vi "Baseplate Locate.vi"() -> ()   [LabVIEW 2020]
uses:
  Classes/Workspace/Workspace.ctl
  Classes/Workspace/Carrier Tray/Assembly Tray.lvclass
  Classes/Controller/Controller.lvclass
  Classes/Routine/Pick and Place/Pick and Place.lvclass
  Classes/Workspace/Fixture.lvclass
panel:
  out "Workspace":T1
  out "Array":dbl[](array[numeric])
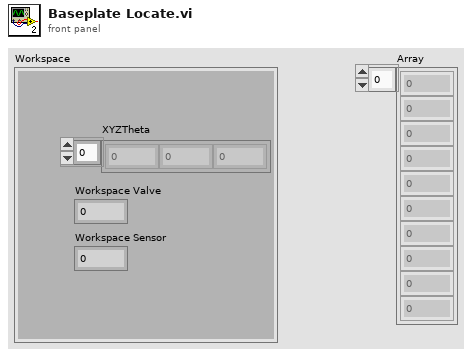
[diagram p1: front panel]
types:
  T1 = typedef "Fixture.lvclass/Workspace.ctl" = cluster{"XYZTheta":dbl[], "Workspace Valve":i32, "Workspace Sensor":i32}
  T2 = typedef "Controller.lvclass/Controllers.ctl" = cluster{"I-O.lvclass":refnum<class "I-O.lvclass">, "Dispenser.lvclass":refnum<class "Dispenser.lvclass">, "Gantry":refnum<k24>}
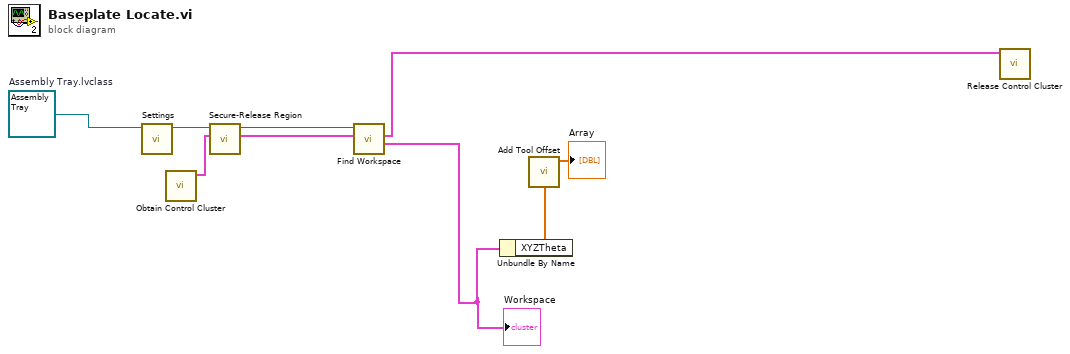
[diagram p0: block diagram]
diagram:
  w9 = refnum<class "Assembly Tray.lvclass"> refnum  # Assembly Tray.lvclass
  n1 = call-dynamic "Settings.vi"("Assembly Tray In"=w9) -> ("Assembly Tray Out"=w8:refnum<class "Assembly Tray.lvclass">)  [unwired: 9 in, 1 out]
  n2 = call "Obtain Control Cluster.vi"() -> ("Control Out"=w6:T2)  [unwired: 11 in]
  n3 = call-dynamic "Secure-Release Region.vi"("Control In"=w6, "Carrier Tray in"=w8) -> ("Control Out"=w5:T2, "Carrier Tray out"=w7:refnum<class "Assembly Tray.lvclass">)  [unwired: 7 in, 1 out]
  n4 = call-dynamic "Find Workspace.vi"("Control In"=w5, "Carrier Tray in"=w7) -> ("Workspace"=w3:T1, "Control Out"=w4:T2)  [unwired: 6 in, 2 out]
  "Workspace" <- w3
  n5 = Unbundle By Name(w3) -> ("XYZTheta"=w2:dbl[])
  n6 = call "Add Tool Offset.vi"("XYZTheta"=w2) -> ("Array"=→"Array":dbl[])  [unwired: 10 in]
  n7 = call "Release Control Cluster.vi"("output cluster"=w4) -> ()  [unwired: 11 in]
